vi "SMO.InstrumentDriver.GenerateNewValueEvent.vi"(8 "error in (no error)":errorcluster, 10 "value":T1, 11 "SMO.InstrumentDriver in":refnum<class "SMO.InstrumentDriver.lvclass">) -> (0 "error out":errorcluster, 3 "SMO.InstrumentDriver out":refnum<class "SMO.InstrumentDriver.lvclass">)   [LabVIEW 2013, in "SMO.InstrumentDriver.lvclass"]
uses:
  SMO.InstrumentDriver.lvclass
  Typedefs/Data.ctl
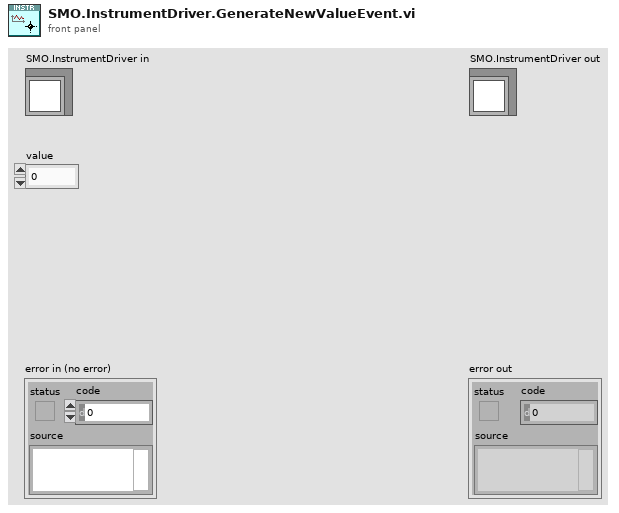
[diagram p1: front panel]
types:
  T1 = typedef "SMO.InstrumentDriver.lvclass/Data.ctl" = dbl
  T2 = typedef "SMO.InstrumentDriver.lvclass/PublicEvents--Cluster.ctl" = cluster{"Value Changed":refnum<user-event>}
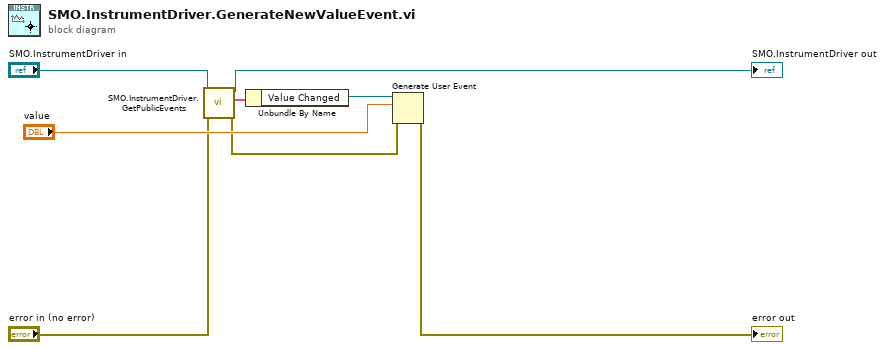
[diagram p0: block diagram]
diagram:
  n1 = call "SMO.InstrumentDriver.GetPublicEvents.vi"("error in (no error)"="error in (no error)", "SMO.Instrument"="SMO.InstrumentDriver in") -> ("error out"=w5:errorcluster, "Instrument Public Events"=w8:T2, "SMO.Instrument out"=→"SMO.InstrumentDriver out":refnum<class "SMO.InstrumentDriver.lvclass">)  [unwired: 7 in]
  n2 = Unbundle By Name(w8) -> ("Value Changed"=w7:refnum<user-event>)
  n3 = Generate User Event(user event=w7, event data cluster="value", error in=w5) -> (error out=→"error out":errorcluster)  [unwired: 1 in, 1 out]
